vi "FromJson.vi"(8 "error in (no error)":errorcluster, 10 "String":string, 11 "Room in":refnum<class "Room.lvclass">) -> (0 "error out":errorcluster, 3 "Room out":refnum<class "Room.lvclass">)   [LabVIEW 2015, in "Room.lvclass"]
uses:
  Room.lvclass
  JsonCluster.ctl
  Room.lvclass/Room.ctl
  Flags/Flags.lvclass
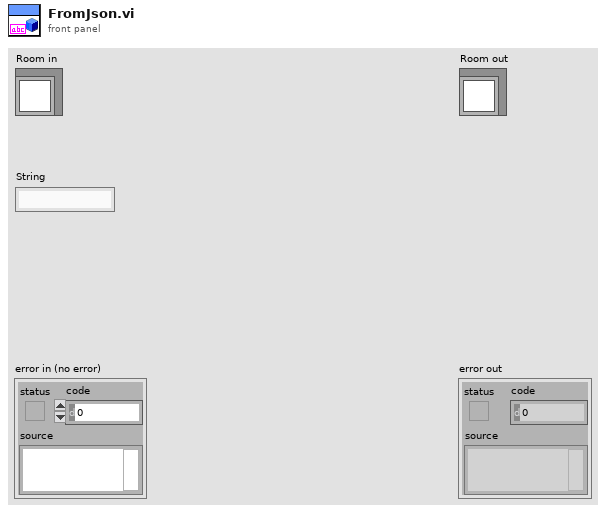
[diagram p1: front panel]
types:
  T1 = typedef "Room.lvclass/JsonCluster.ctl" = cluster{"Flags":string, "BedVacant":bool, "InRoomPersonnel":string[], "RoomRequests":string[], "Beacon Id":string, "Bed URL":string}
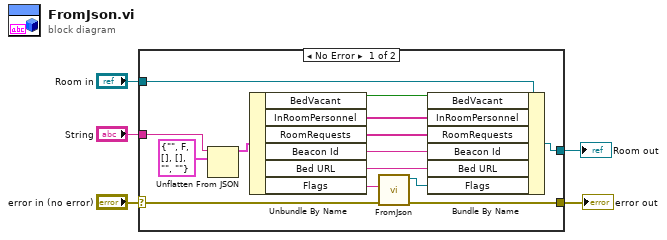
[diagram p0: block diagram]
diagram:
  n1 = case shown="No Error" "error in (no error)" {
    selector: "error in (no error)" -> [w12 w21]
    tunnel: [w11 w21] -> w4
    tunnel: [w16 w20] -> w2
    tunnel: "Room in" -> [w17 w20]
    tunnel: "String" -> [w19 _]
    frame No Error {
      n2 = Unflatten From JSON(JSON string=w19, type and defaults=T1 {"Flags"="", "BedVacant"=FALSE, "InRoomPersonnel"=[], "RoomRequests"=[], "Beacon Id"="", "Bed URL"=""} ("Room")) -> (value=w15:T1)  [unwired: 5 in, 1 out]
      n3 = Unbundle By Name(w15) -> ("BedVacant"=w7:bool, "InRoomPersonnel"=w8:string[], "RoomRequests"=w9:string[], "Beacon Id"=w10:string, "Bed URL"=w6:string, "Flags"=w14:string)
      n4 = call "FromJson.vi"("error in (no error)"=w12, "String"=w14) -> ("error out"=w11:errorcluster, "Flags out"=w13:refnum<class "Flags.lvclass">)  [unwired: 8 in]
      n5 = Bundle By Name(cluster=w17, "BedVacant"=w7, "InRoomPersonnel"=w8, "RoomRequests"=w9, "Beacon Id"=w10, "Bed URL"=w6, "Flags"=w13) -> (w16:refnum<class "Room.lvclass">)
    }
    frame Error {
    }
  }
  "error out" <- w4
  "Room out" <- w2
